vi "Get LVAddons Directory.vi"(8 "error in":errorcluster) -> (0 "error out":errorcluster, 3 "LVAddons Directory":string)   [LabVIEW 2019, in "SEECD System Explorer.lvlib"]
uses:
  <vilib>/registry/registry.llb/Registry RtKey.ctl
  <vilib>/registry/registry.llb/Registry SAM.ctl
  SEECD System Explorer.lvlib
  <vilib>/registry/registry.llb/Read Registry Value Simple STR.vi
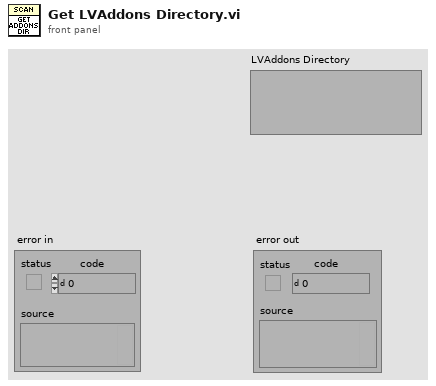
[diagram p1: front panel]
types:
  T1 = typedef "Registry SAM.ctl" = enum32{"KEY_QUERY_VALUE", "KEY_SET_VALUE", "KEY_CREATE_SUB_KEY", "KEY_ENUMERATE_SUB_KEYS", "KEY_NOTIFY", "KEY_CREATE_LINK", "KEY_READ", "KEY_WRITE", "KEY_ALL_ACCESS", "KEY_READ | KEY_WRITE"}
  T2 = typedef "Registry RtKey.ctl" = enum32{"HKEY_CLASSES_ROOT", "HKEY_CURRENT_USER", "HKEY_LOCAL_MACHINE", "HKEY_USERS", "HKEY_PERFORMANCE_DATA", "HKEY_CURRENT_CONFIG", "HKEY_DYN_DATA"}
  T3 = typedef "Registry refnum.ctl" = refnum<k1>
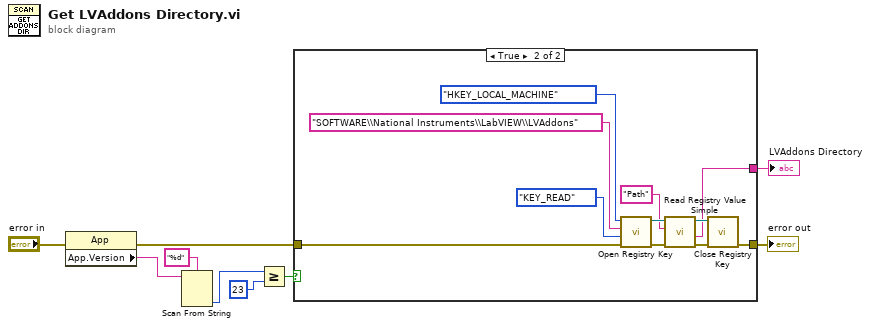
[diagram p0: block diagram]
diagram:
  n1 = property class="App"(error in="error in") -> (error out=w2:errorcluster, "App.Version"=w6:string)  [unwired: 1 in, 1 out]
  n2 = Scan From String(format string="%d", input string=w6) -> (output 1=w4:i32)  [unwired: 3 in, 3 out]
  n3 = Greater Or Equal?(x=w4, y=23) -> (x >= y?=w1:bool)
  n4 = case shown="True" w1 {
    tunnel: [w10 w15] -> w9
    tunnel: [_ w13] -> w8
    tunnel: w2 -> [w10 w11]
    frame False {
    }
    frame True {
      n5 = call <vilib>:"Open Registry Key.vi"("error in (no error)"=w11, "security access mask (KEY_READ | KEY_WRITE)"=Registry_SAM."KEY_READ", "subkey"="SOFTWARE\\National Instruments\\LabVIEW\\LVAddons", "root key (HKEY_LOCAL_MACHINE)"=Registry_RtKey."HKEY_LOCAL_MACHINE") -> ("error out"=w17:errorcluster, "refnum out"=w16:T3)  [unwired: 6 in]
      n6 = call-poly <vilib>:"Read Registry Value Simple.vi"("error in (no error)"=w17, "value"="Path", "refnum"=w16) -> ("error out"=w21:errorcluster, "String/Binary data"=w13:string, "refnum out"=w20:T3)  [unwired: 3 in, 1 out]
      n7 = call <vilib>:"Close Registry Key.vi"("error in (no error)"=w21, "refnum"=w20) -> ("error out"=w15:errorcluster)  [unwired: 5 in]
    }
  }
  "error out" <- w9
  "LVAddons Directory" <- w8
